vi "FunctDataMgr.Reset Data.vi"(8 "error in (no error)":errorcluster, 11 "FunctDataMgr in":refnum<class "FunctDataMgr.lvclass">) -> (0 "error out":errorcluster, 3 "FunctDataMgr out":refnum<class "FunctDataMgr.lvclass">)   [LabVIEW 2018, in "FunctDataMgr.lvclass"]
uses:
  FunctDataMgr.lvclass
  TestExec/TestExec.Local Result Data.ctl
  Results/Result.Attribute.ctl
  Results/Result.Measurement and Attribute Item Status.ctl
  Results/Result.Numeric.ctl
  Results/Result.Limit Type.ctl
  Results/Result XML/TestResult.SW Item.ctl
  Reports/Report.Result FileDataObject.ctl
  Results/Result.Measurement Item.ctl
  <vilib>/KATE/SeqMgr/SeqMgr.Result Info.ctl
  <vilib>/KATE/SeqMgr/SeqMgr.Result State Enum.ctl
  FunctDataMgr.lvclass/FunctDataMgr.ctl
  <vilib>/KATE/SeqMgr/SeqMgr.lvlib
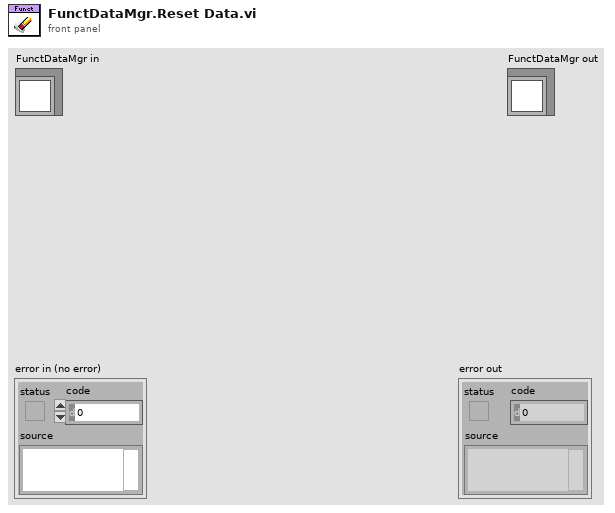
[diagram p1: front panel]
types:
  T1 = typedef "KATE_Lib.lvlib/SeqMgr.lvlib/SeqMgr.Result Info.ctl" = cluster{"State":T2, "Code":i32, "Description":string}
  T2 = typedef "KATE_Lib.lvlib/SeqMgr.lvlib/SeqMgr.Result State Enum.ctl" = enum16{"None", "Passing", "Failing", "PASS", "FAIL", "ABORT", "ERROR"}
  T3 = cluster{"Sequence":string, "Mode":string, "SN":string, "StartTime":timestamp, "Pos":i32}
  T4 = typedef "TestExec.Local Result Data.ctl" = cluster{"Attr":T5[], "Num":T7[], "UUT Props":string[][], "Vars":string[][], "SW Items":T9[], "Error":errorcluster, "Step":i32, "FileObjs":T10[], "MeasData":T11[]}
  T5 = typedef "Result.Attribute.ctl" = cluster{"Cnt":i32, "Step":string, "Category":string, "Name":string, "Value":string, "Status":T6, "Code":i32, "Desc":string, "Time":timestamp}
  T6 = typedef "Result.Measurement and Attribute Item Status.ctl" = i32
  T7 = typedef "Result.Numeric.ctl" = cluster{"Cnt":i32, "Step":string, "Category":string, "Name":string, "Value":dbl, "Units":string, "LimType":T8, "LL":dbl, "UL":dbl, "Status":T6, "Code":i32, "Desc":string, "Time":timestamp}
  T8 = typedef "Result.Limit Type.ctl" = enum16{"None", "EQ", "NE", "GT", "LT", "GE", "LE", "GTLT", "GELE", "GELT", "GTLE", "LTGT", "LEGE", "LEGT", "LTGE", "Contains", "NotContains"}
  T9 = typedef "TestResult.SW Item.ctl" = cluster{"Name":string, "PN":string, "Version":string, "Note":string}
  T10 = typedef "Report.Result FileDataObject.ctl" = cluster{"Cnt":i32, "Step":string, "Category":string, "Name":string, "Type":string, "File Name":string, "Time":string, "Path":path}
  T11 = typedef "Result.Measurement Item.ctl" = cluster{"Cnt":i32, "Step":string, "Category":string, "Name":string, "Value":string, "Units":string, "LimType":string, "LL":string, "UL":string, "Status":T6, "Code":i32, "Desc":string, "Time":timestamp}
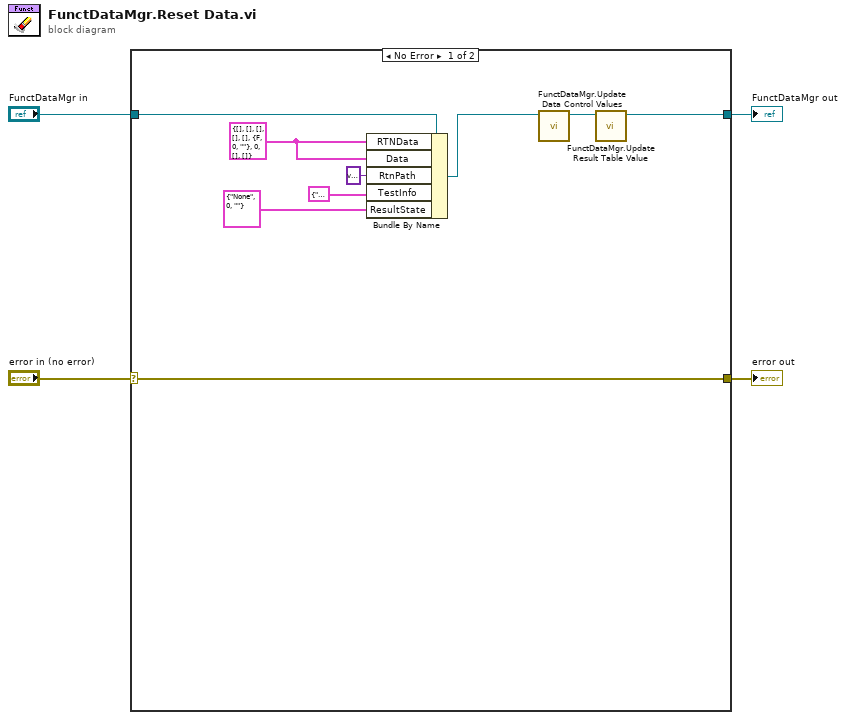
[diagram p0: block diagram]
diagram:
  n1 = case shown="No Error" "error in (no error)" {
    selector: "error in (no error)" -> [w13 w15]
    tunnel: [w13 w15] -> w3
    tunnel: [w6 w14] -> w1
    tunnel: "FunctDataMgr in" -> [w12 w14]
    frame No Error {
      w11 = T4 {"Attr"=[], "Num"=[], "UUT Props"=[], "Vars"=[], "SW Items"=[], "Error"={"status"=FALSE, "code"=0, "source"=""}, "Step"=0, "FileObjs"=[], "MeasData"=[]} ("RTN Data")
      n2 = Bundle By Name(cluster=w12, "RTNData"=w11, "Data"=w11, "RtnPath"=variant, "TestInfo"=T3 {"Sequence"="", "Mode"="", "SN"="", "StartTime"=timestamp(0 s since 1904-01-01), "Pos"=0}, "ResultState"=T1 {"State"=enum."None", "Code"=0, "Description"=""} ("Result Info")) -> (w7:refnum<class "FunctDataMgr.lvclass">)
      n3 = call "FunctDataMgr.Update Data Control Values.vi"("FunctDataMgr in"=w7) -> ("FunctDataMgr out"=w8:refnum<class "FunctDataMgr.lvclass">)  [unwired: 9 in, 1 out]
      n4 = call "FunctDataMgr.Update Result Table Value.vi"("FunctDataMgr in"=w8) -> ("FunctDataMgr out"=w6:refnum<class "FunctDataMgr.lvclass">)  [unwired: 9 in, 1 out]
    }
    frame Error {
    }
  }
  "error out" <- w3
  "FunctDataMgr out" <- w1
